vi "iow28_adc_singleshot.vi"() -> ()   [LabVIEW 2011]
panel:
  out "arrayout":u8[](array[numeric]) format="%x"
  out "Error Read":errorcluster caption="error"
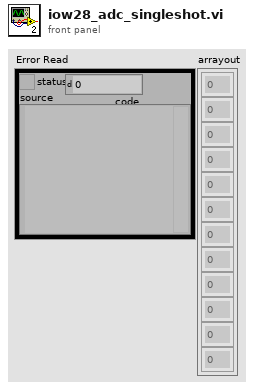
[diagram p1: front panel]
types:
  T1 = typedef "IOWarrior_Handle.ctl" = cluster{"Handle":u32, "Serial Number":string, "type of Warrior":T2, "Root Handle":bool, "Revision":u16}
  T2 = typedef "IOWarrior_Type.ctl" = enum16{"invalid", "IOW24", "IOW40", "IOW56", "IOPV1", "IOPV2", "IOW28"}
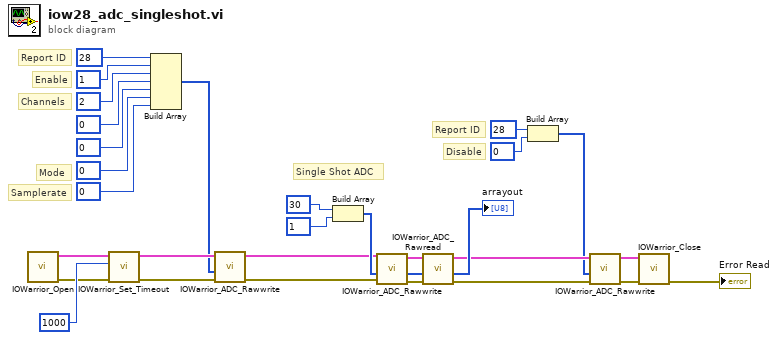
[diagram p0: block diagram]
diagram:
  # "Disable"
  # "Report ID"
  # "Single Shot ADC"
  # "Samplerate"
  # "Mode"
  # "Channels"
  # "Enable"
  # "Report ID"
  n1 = call "IOWarrior_Open.vi"() -> ("err out"=w23:errorcluster, "IOWarriorHandle"=w24:T1)  [unwired: 9 in, 1 out]
  n2 = call "IOWarrior_Set_Timeout.vi"("err in"=w23, "timeout_ms(1000)"=1000, "devHandle"=w24) -> ("err out"=w19:errorcluster, "devHandleout"=w18:T1)  [unwired: 6 in, 1 out]
  n3 = Build Array(u8 28, u8 1, u8 2, u8 0, u8 0, u8 0, u8 0) -> (w17:u8[])
  n4 = call "IOWarrior_ADC_Rawwrite.vi"("err in"=w19, "Array_in"=w17, "devHandle"=w18) -> ("err out"=w8:errorcluster, "devHandleout"=w12:T1)  [unwired: 6 in, 1 out]
  n5 = Build Array(u8 30, u8 1) -> (w15:u8[])
  n6 = call "IOWarrior_ADC_Rawwrite.vi"("err in"=w8, "Array_in"=w15, "devHandle"=w12) -> ("err out"=w9:errorcluster, "array_out"=w10:u8[], "devHandleout"=w11:T1)  [unwired: 6 in]
  n7 = call "IOWarrior_ADC_Rawread.vi"("err in"=w9, "array"=w10, "devHandle"=w11) -> ("err out"=w2:errorcluster, "arrayout"=→"arrayout":u8[], "devHandleout"=w3:T1)  [unwired: 6 in]
  n8 = Build Array(u8 28, u8 0) -> (w1:u8[])
  n9 = call "IOWarrior_ADC_Rawwrite.vi"("err in"=w2, "Array_in"=w1, "devHandle"=w3) -> ("err out"=w4:errorcluster, "devHandleout"=w5:T1)  [unwired: 6 in, 1 out]
  n10 = call "IOWarrior_Close.vi"("err in"=w4, "devHandle"=w5) -> ("err out"=→"Error Read":errorcluster)  [unwired: 8 in, 1 out]
